vi "to_json.vi"(8 "error in":errorcluster, 11 "timestampType in":refnum<class "timestampType.lvclass">) -> (0 "error out":errorcluster, 2 "json":string, 3 "timestampType out":refnum<class "timestampType.lvclass">)   [LabVIEW 2020, in "timestampType.lvclass"]
uses:
  timestampType.lvclass
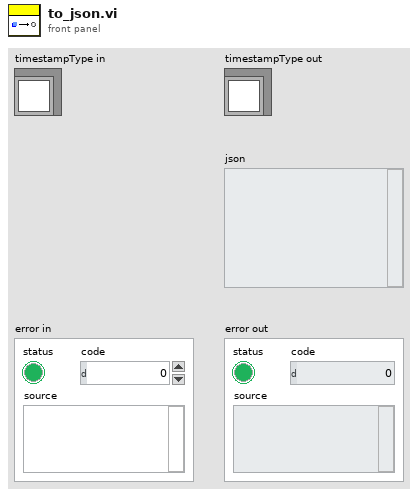
[diagram p1: front panel]
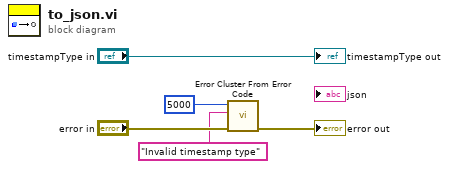
[diagram p0: block diagram]
diagram:
  n1 = call <vilib>:"Error Cluster From Error Code.vi"("error in (no error)"="error in", "error message (\"\")"="Invalid timestamp type" ("error message (\"\")"), "error code (0)"=5000) -> ("error out"=→"error out":errorcluster)  [unwired: 6 in]
  "timestampType out" <- "timestampType in"
